vi "Teleop.vi"(10 "Match Info":T1={"Autonomous Elapsed Seconds"=0.0, "TeleOp Elapsed Seconds"=0.0, "Disabled Elapsed Seconds"=0.0, "Visited Autonomous"=FALSE, "Visited TeleOp"=FALSE, "Visited Disabled"=FALSE, "Autonomous Settings"={"Autonomous Style"=enum."Independent", "VI Refnum"=refnum}}, 11 "Call Context":T2) -> ()   [LabVIEW 2015]
doc: "This VI is called for each TeleOp packet received from the DS where the robot is not disabled. It is often used to read from the joysticks and update I/O or to update setpoints for timed control loops. It should complete and return within 20 milliseconds or it may miss DS packets."
uses:
  <vilib>/Rock Robotics/WPI/DriverStation/WPI_DriverStationDerivedRobotMode.ctl
  <vilib>/Rock Robotics/WPI/DriverStation/WPI_DriverStationMatch Info.ctl
  <vilib>/Rock Robotics/Network Tables/NT Read Boolean.vi
  <vilib>/Rock Robotics/Network Tables/NT Read Number.vi
  <vilib>/Rock Robotics/WPI/Utilities/WPI_GetSetVariantRefNum.vi
  Robot Global Data.vi
  <vilib>/Rock Robotics/Network Tables/NT Write Boolean Array.vi
  <vilib>/Rock Robotics/Network Tables/NT Write Numeric Array.vi
  <vilib>/Rock Robotics/WPI/RobotDrive/WPI_RobotDriveMecanumDrive_Cartesian.vi
panel:
  out "Sample Slider 0":dbl(slide) scale=0.0..5.0
  out "Sample Boolean 1":bool
  out "Sample Boolean 0":bool
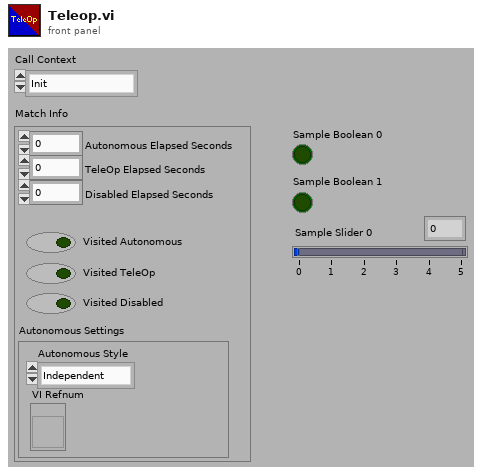
[diagram p1: front panel]
types:
  T1 = typedef "WPI_DriverStationMatch Info.ctl" = cluster{"Autonomous Elapsed Seconds":dbl, "TeleOp Elapsed Seconds":dbl, "Disabled Elapsed Seconds":dbl, "Visited Autonomous":bool, "Visited TeleOp":bool, "Visited Disabled":bool, "Autonomous Settings":cluster{"Autonomous Style":enum16{"Iterative", "Independent"}, "VI Refnum":refnum<vi>}}
  T2 = typedef "WPI_DriverStationDerivedRobotMode.ctl" = enum16{"Init", "Execute", "Stop"}
  T3 = typedef "WPI_JoystickDevRef.ctl" = cluster{"Device":T4}
  T4 = typedef "WPI_JoystickDeviceEnum.ctl" = enum16{"USB 0", "USB 1", "USB 2", "USB 3", "USB 4", "USB 5"}
  T5 = typedef "WPI_RobotDriveDevRef.ctl" = cluster{"DevStatus":errorcluster, "Motors[]":T6[], "Square Inputs":bool, "Max Output":dbl}
  T6 = typedef "WPI_MotorControlDeviceRef.ctl" = cluster{"DeviceStatus":errorcluster, "Type":T7, "PWM":cluster{"PWM Channel":T8, "DeadBand":T9}, "CAN":cluster{"Device Number":u8, "Control Mode":T10, "Semaphore":T11, "Max Vout":dbl, "TalonSRX Control Mode":T12}, "Invert":bool}
  T7 = typedef "WPI_MotorControlType.ctl" = enum16{"PWM", "CAN", "CANTalonSRX"}
  T8 = typedef "FPGA_DIOPWMChannel.ctl" = enum8{"PWM 0", "PWM 1", "PWM 2", "PWM 3", "PWM 4", "PWM 5", "PWM 6", "PWM 7", "PWM 8", "PWM 9", "PWM MXP 0", "PWM MXP 1", "PWM MXP 2", "PWM MXP 3", "PWM MXP 4", "PWM MXP 5", "PWM MXP 6", "PWM MXP 7", "PWM MXP 8", "PWM MXP 9", "Invalid"}
  T9 = typedef "WPI_PWMDeadband.ctl" = cluster{"Name":string, "maxPositivePwm":i32, "minPositivePwm":i32, "centerPwm":i32, "maxNegativePwm":i32, "minNegativePwm":i32, "angularRange":u16}
  T10 = typedef "WPI_CANJaguar_ControlMode.ctl" = enum8{"Percent VBus", "Current", "Speed", "Position", "Voltage"}
  T11 = typedef "Semaphore RefNum" = refnum<k1>
  T12 = typedef "WPI_CANTalonSRX_APIControlMode.ctl" = enum8{"Percent VBus", "Speed", "Position", "Slave", "Unchanged / Invalid", "Voltage Compensation", "Current", "Motion Profile"}
  T13 = cluster{"Buttons[0]":bool, "Buttons[1]":bool, "Buttons[2]":bool, "Buttons[3]":bool, "Buttons[4]":bool, "Buttons[5]":bool, "Buttons[6]":bool, "Buttons[7]":bool, "Buttons[8]":bool}
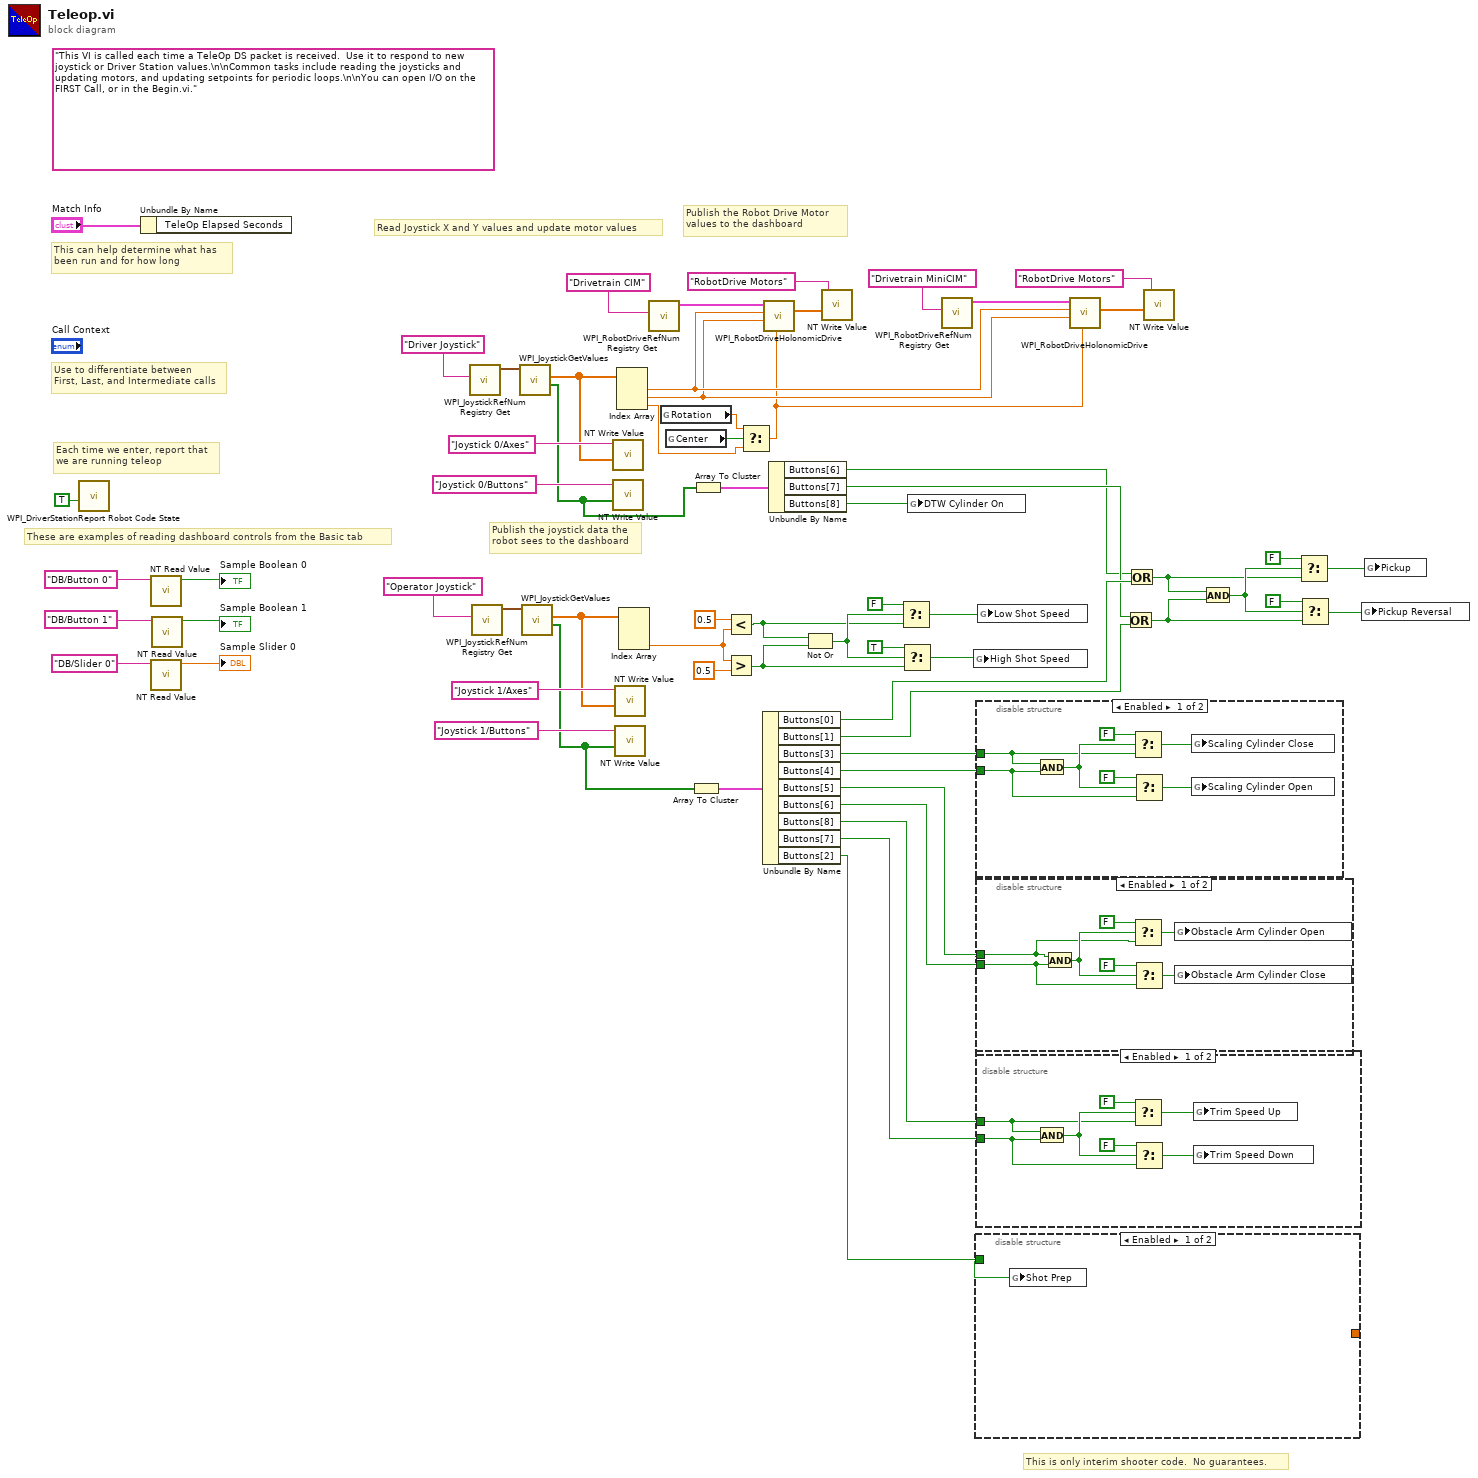
[diagram p0: block diagram]
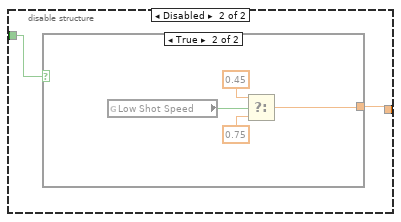
[diagram p2: hidden frame]
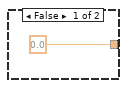
[diagram p3: hidden frame]
diagram:
  (unwired) "This VI is called each time a TeleOp DS packet is received.  Use it to respond to new joystick or Driver Station values.\n\nCommon tasks include reading the joysticks and updating motors, and updating setpoints for periodic loops.\n\nYou can open I/O on the FIRST Call, or in the Begin.vi."
  # "This is only interim shooter code.  No guarantees."
  # "Publish the Robot Drive Motor\nvalues to the dashboard"
  # "Publish the joystick data the\nrobot sees to the dashboard"
  # "Read Joystick X and Y values and update motor values"
  # "These are examples of reading dashboard controls from the Basic tab"
  # "Each time we enter, report that\nwe are running teleop"
  # "Use to differentiate between\nFirst, Last, and Intermediate calls"
  # "This can help determine what has\nbeen run and for how long"
  n1 = call <vilib>:"WPI_DriverStationReport Robot Code State.vi"("TeleOp"=TRUE ("Autonomous")) -> ()  [unwired: 10 in, 1 out]
  n2 = Unbundle By Name("Match Info") -> ()  [unwired: 1 out]
  n3 = call-poly <vilib>:"NT Read Value.vi"("Name"="DB/Button 0" ("refnum name")) -> ("Boolean"=→"Sample Boolean 0":bool)  [unwired: 9 in, 1 out]
  n4 = call-poly <vilib>:"NT Read Value.vi"("Name"="DB/Slider 0" ("refnum name")) -> ("Numeric"=→"Sample Slider 0":dbl)  [unwired: 9 in, 1 out]
  n5 = call-poly <vilib>:"NT Read Value.vi"("Name"="DB/Button 1" ("refnum name")) -> ("Boolean"=→"Sample Boolean 1":bool)  [unwired: 9 in, 1 out]
  n6 = call <vilib>:"WPI_JoystickRefNum Registry Get.vi"("refnum name"="Driver Joystick") -> ("JoystickDevRef"=w53:T3)  [unwired: 1 in, 9 out]
  n7 = call <vilib>:"WPI_JoystickRefNum Registry Get.vi"("refnum name"="Operator Joystick") -> ("JoystickDevRef"=w46:T3)  [unwired: 1 in, 9 out]
  n8 = call <vilib>:"WPI_JoystickGetValues.vi"("JoystickDevRef"=w53) -> ("Buttons"=w51:bool[], "Axes"=w55:dbl[])  [unwired: 6 in, 3 out]
  n9 = call <vilib>:"WPI_JoystickGetValues.vi"("JoystickDevRef"=w46) -> ("Buttons"=w44:bool[], "Axes"=w48:dbl[])  [unwired: 6 in, 3 out]
  n10 = call-poly <vilib>:"NT Write Value.vi"("Numeric Array"=w55, "Name"="Joystick 0/Axes") -> ()  [unwired: 9 in, 1 out]
  n11 = call-poly <vilib>:"NT Write Value.vi"("Boolean Array"=w51, "Name"="Joystick 0/Buttons") -> ()  [unwired: 9 in, 1 out]
  n12 = call-poly <vilib>:"NT Write Value.vi"("Numeric Array"=w48, "Name"="Joystick 1/Axes") -> ()  [unwired: 9 in, 1 out]
  n13 = call-poly <vilib>:"NT Write Value.vi"("Boolean Array"=w44, "Name"="Joystick 1/Buttons") -> ()  [unwired: 9 in, 1 out]
  n14 = Index Array(array=w55) -> (element #1=w43:dbl, element #2=w42:dbl, element #3=w3:dbl)  [unwired: 3 in]
  n15 = Index Array(array=w48) -> (element #3=w34:dbl)  [unwired: 3 in, 2 out]
  n16 = call <vilib>:"WPI_RobotDriveRefNum Registry Get.vi"("refnum name"="Drivetrain CIM") -> ("RobotDriveDevRef"=w28:T5)  [unwired: 1 in, 9 out]
  n17 = global read "Robot Global Data.vi" "Rotation"() -> (w1:dbl)
  n18 = global read "Robot Global Data.vi" "Center"() -> (w2:bool)
  n19 = Array To Cluster(array=w44) -> (cluster=w45:T13)
  n20 = Array To Cluster(array=w51) -> (cluster=w52:T13)
  n21 = Less?(x=0.5 ("y"), y=w34) -> (x < y?=w33:bool)
  n22 = Greater?(x=w34, y=0.5) -> (0:w32:bool)
  n23 = Select(t=w1, s=w2, f=w3) -> (s? t:f=w4:dbl)
  n24 = Unbundle By Name(w45) -> ("Buttons[0]"=w13:bool, "Buttons[1]"=w14:bool, "Buttons[3]"=w41:bool, "Buttons[4]"=w40:bool, "Buttons[5]"=w8:bool, "Buttons[6]"=w7:bool, "Buttons[8]"=w6:bool, "Buttons[7]"=w5:bool, "Buttons[2]"=w9:bool)
  n25 = call-poly <vilib>:"WPI_RobotDriveHolonomicDrive.vi"("Rotation"=w4, "Y"=w42, "X"=w43, "RobotDriveDevRef"=w28) -> ("Motor Values"=w26:dbl[])  [unwired: 5 in, 2 out]
  n26 = Unbundle By Name(w52) -> ("Buttons[6]"=w11:bool, "Buttons[7]"=w12:bool, "Buttons[8]"=w10:bool)
  n27 = Not Or(1:w32, 2:w33) -> (0:w37:bool)
  n28 = call-poly <vilib>:"NT Write Value.vi"("Numeric Array"=w26, "Name"="RobotDrive Motors") -> ()  [unwired: 9 in, 1 out]
  n29 = Select(t=FALSE, s=w37, f=w33) -> (s? t:f=w30:bool)
  n30 = Select(t=TRUE, s=w37, f=w32) -> (s? t:f=w31:bool)
  n31 = global write "Robot Global Data.vi" "DTW Cylinder On"(w10) -> ()
  n32 = call <vilib>:"WPI_RobotDriveRefNum Registry Get.vi"("refnum name"="Drivetrain MiniCIM") -> ("RobotDriveDevRef"=w24:T5)  [unwired: 1 in, 9 out]
  n33 = global write "Robot Global Data.vi" "High Shot Speed"(w31) -> ()
  n34 = disable-structure shown="Enabled" {
    disable-tunnel: w9 -> [w66 w68]
    disable-tunnel: [_ w67] -> _
    frame Enabled {
      n35 = global write "Robot Global Data.vi" "Shot Prep"(w66) -> ()
    }
    frame Disabled {
      n36 = case shown="True" w68 {
        tunnel: [0.0 w70] -> w67
        frame False {
        }
        frame True {
          n37 = global read "Robot Global Data.vi" "Low Shot Speed"() -> (w73:bool)
          n38 = Select(t=0.45, s=w73, f=0.75) -> (s? t:f=w70:dbl)
        }
      }
    }
  }
  n39 = disable-structure shown="Enabled" {
    disable-tunnel: w41 -> [w79 _]
    disable-tunnel: w40 -> [w78 _]
    frame Enabled {
      n40 = And(x=w79, y=w78) -> (x .and. y?=w80:bool)
      n41 = Select(t=FALSE, s=w80, f=w79) -> (s? t:f=w74:bool)
      n42 = Select(t=FALSE, s=w80, f=w78) -> (s? t:f=w75:bool)
      n43 = global write "Robot Global Data.vi" "Scaling Cylinder Close"(w74) -> ()
      n44 = global write "Robot Global Data.vi" "Scaling Cylinder Open"(w75) -> ()
    }
    frame Disabled {
    }
  }
  n45 = disable-structure shown="Enabled" {
    disable-tunnel: w7 -> [w82 _]
    disable-tunnel: w8 -> [w81 _]
    frame Enabled {
      n46 = And(x=w81, y=w82) -> (x .and. y?=w87:bool)
      n47 = Select(t=FALSE, s=w87, f=w81) -> (s? t:f=w83:bool)
      n48 = Select(t=FALSE, s=w87, f=w82) -> (s? t:f=w84:bool)
      n49 = global write "Robot Global Data.vi" "Obstacle Arm Cylinder Open"(w83) -> ()
      n50 = global write "Robot Global Data.vi" "Obstacle Arm Cylinder Close"(w84) -> ()
    }
    frame Disabled {
    }
  }
  n51 = disable-structure shown="Enabled" {
    disable-tunnel: w6 -> [w93 _]
    disable-tunnel: w5 -> [w92 _]
    frame Enabled {
      n52 = And(x=w93, y=w92) -> (x .and. y?=w94:bool)
      n53 = Select(t=FALSE, s=w94, f=w93) -> (s? t:f=w88:bool)
      n54 = Select(t=FALSE, s=w94, f=w92) -> (s? t:f=w89:bool)
      n55 = global write "Robot Global Data.vi" "Trim Speed Up"(w88) -> ()
      n56 = global write "Robot Global Data.vi" "Trim Speed Down"(w89) -> ()
    }
    frame Disabled {
    }
  }
  n57 = global write "Robot Global Data.vi" "Low Shot Speed"(w30) -> ()
  n58 = call-poly <vilib>:"WPI_RobotDriveHolonomicDrive.vi"("Rotation"=w4, "Y"=w42, "X"=w43, "RobotDriveDevRef"=w24) -> ("Motor Values"=w23:dbl[])  [unwired: 5 in, 2 out]
  n59 = Or(x=w12, y=w14) -> (x .or. y?=w15:bool)
  n60 = Or(x=w11, y=w13) -> (x .or. y?=w16:bool)
  n61 = call-poly <vilib>:"NT Write Value.vi"("Numeric Array"=w23, "Name"="RobotDrive Motors") -> ()  [unwired: 9 in, 1 out]
  n62 = And(x=w16, y=w15) -> (x .and. y?=w21:bool)
  n63 = Select(t=FALSE, s=w21, f=w16) -> (s? t:f=w18:bool)
  n64 = Select(t=FALSE, s=w21, f=w15) -> (s? t:f=w17:bool)
  n65 = global write "Robot Global Data.vi" "Pickup Reversal"(w17) -> ()
  n66 = global write "Robot Global Data.vi" "Pickup"(w18) -> ()
